vi "ICM Write General Parameters.vi"(9 "Re-Init?":bool, 10 "ICM File In":path, 11 "ICM General Parameters":T1 {"Time" format="%<%H:%M:%S>t"; "Date" format="%<%Y/%m/%d>T"; "Version" format="%.1g"}) -> (0 "error out":errorcluster)   [LabVIEW 2018]
doc: "ICM Write General Parameters.vi\n\nThis VI is used to write the General Parameters to the ICM Configuration file.\n\nInstrument Communication Module Version 1.0\nAugust, 2017 Original Code Consulting David Thomson\n www.originalcode.com"
uses:
  Controls/ICM General Parameters.ctl
panel:
  # "The values for these\nparameters are generally\nset by the ICM system and\nneed not be edited directly."
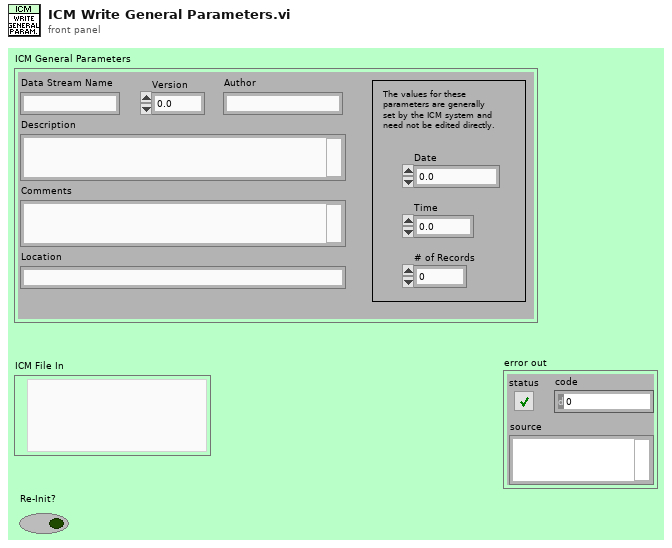
[diagram p1: front panel]
types:
  T1 = typedef "ICM General Parameters.ctl" = cluster{"Data Stream Name":string, "Version":sgl, "Author":string, "Description":string, "Comments":string, "Date":dbl, "Time":dbl, "Location":string, "# of Records":i32}
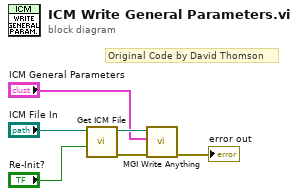
[diagram p0: block diagram]
diagram:
  # "Original Code by David Thomson"
  n1 = call "Get ICM File.vi"("Re-Init?"="Re-Init?", "ICM File In"="ICM File In") -> ("error out"=w6:errorcluster, "ICM File"=w5:path)  [unwired: 8 in]
  n2 = call <userlib>:"MGI Write Anything.vi"("Error In"=w6, "Anything"="ICM General Parameters", "Path (dialog)"=w5) -> ("Error Out"=→"error out":errorcluster)  [unwired: 6 in, 2 out]
